vi "DelayLeft.vi"(2 "sample in":fxp<+/-,25,16>, 3 "n":i64) -> (0 "SampleOut":fxp<+/-,25,16>)   [LabVIEW 2016]
uses:
  <vilib>/rvi/Emulation/niFpgaGetClockAttributes.vi
  <vilib>/rvi/Emulation/niFpgaSctlEmulationGetInTimedLoop.vi
  <vilib>/rvi/Emulation/niFpgaEmulationReportErrorSimple.vi
  Global 1.vi
  <vilib>/rvi/Memory/Memory_Emulation/nirvimemoryFastEmulation.vi
  <vilib>/rvi/Memory/Memory_Emulation/nirvimemoryEmulation.vi
  <vilib>/rvi/Emulation/niFpgaEmulationIsFPGAContextNoSignature.vi
  <vilib>/rvi/DataTransferAndStorage/Container/Common/niFpgaContainerGetUniqueNameForEmu.vi
  <vilib>/rvi/Emulation/niFpgaProcessEmulError.vi
  <vilib>/rvi/errors/nirviReportUnexpectedCaseInternalError (U32).vi
  <vilib>/rvi/Emulation/niFpgaCriticalErrorInLSC.vi
  <vilib>/rvi/DataTransferAndStorage/Container/XNode/niFpgaContainer.xnode
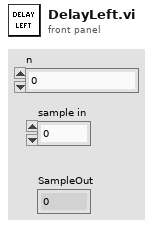
[diagram p1: front panel]
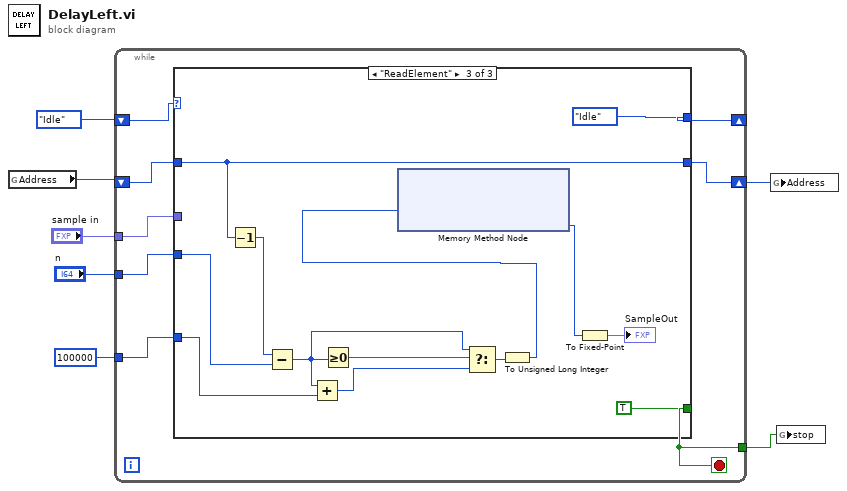
[diagram p0: block diagram]
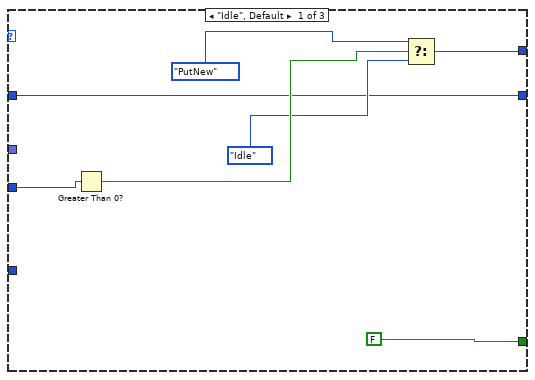
[diagram p2: hidden frame]
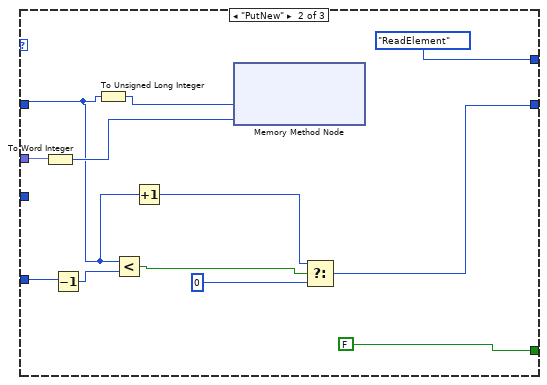
[diagram p3: hidden frame]
diagram:
  n1 = global read "Global 1.vi" "Address"() -> (w6:i64)
  n2 = while {
    shift-right: [w13] -> _
    shift-left: enum16{"Idle", "PutNew", "ReadElement"}."Idle" -> [w15]
    shift-right: [w12] -> w4
    shift-left: w6 -> [w11]
    tunnel: "n" -> [w14]
    tunnel: "sample in" -> [w10]
    tunnel: i64 100000 -> [w9]
    tunnel: [w8] -> w1
    stop <- w8 stop-if-true
    n3 = case shown="\"ReadElement\"" w15 {
      tunnel: w14 -> [w22 _ w45]
      tunnel: [w18 enum16{"Idle", "PutNew", "ReadElement"}."ReadElement" enum16{"Idle", "PutNew", "ReadElement"}."Idle"] -> w13
      tunnel: [w17 w29 w44] -> w12
      tunnel: w11 -> [w17 w23 w44]
      tunnel: w10 -> [_ w26 _]
      tunnel: w9 -> [_ w34 w43]
      tunnel: [FALSE FALSE TRUE] -> w8
      frame "Idle", Default {
        n4 = Greater Than 0?(x=w22) -> (x > 0?=w21:bool)
        n5 = Select(t=enum16{"Idle", "PutNew", "ReadElement"}."PutNew", s=w21, f=enum16{"Idle", "PutNew", "ReadElement"}."Idle") -> (s? t:f=w18:enum16{"Idle", "PutNew", "ReadElement"})
      }
      frame "PutNew" {
        n6 = To Word Integer(number=w26) -> (16bit integer=w25:i16)
        n7 = Decrement(x=w34) -> (x-1=w33:i64)
        n8 = To Unsigned Long Integer(number=w23) -> (unsigned 32bit integer=w24:u32)
        n9 = Less?(x=w23, y=w33) -> (x < y?=w31:bool)
        n10 = Increment(x=w23) -> (x+1=w32:i64)
        n11 = xnode ("Memory Method Node")("Address"=w24, "Data"=w25) -> ()  [unwired: 1 in, 1 out]
        n12 = Select(t=w32, s=w31, f=u32 0) -> (s? t:f=w29:i64)
      }
      frame "ReadElement" {
        n13 = Decrement(x=w44) -> (x-1=w46:i64)
        n14 = Subtract(x=w46, y=w45) -> (x-y=w37:i64)
        n15 = Add(x=w37, y=w43) -> (x+y=w41:i64)
        n16 = Greater Or Equal To 0?(x=w37) -> (x >= 0?=w42:bool)
        n17 = Select(t=w37, s=w42, f=w41) -> (s? t:f=w36:i64)
        n18 = To Unsigned Long Integer(number=w36) -> (unsigned 32bit integer=w35:u32)
        n19 = xnode ("Memory Method Node")("Address"=w35) -> ("Data"=w39:i16)  [unwired: 1 in, 1 out]
        n20 = To Fixed-Point(number=w39) -> (fixed-point=→"SampleOut":fxp<+/-,25,16>)  [unwired: 1 in]
      }
    }
  }
  n21 = global write "Global 1.vi" "Address"(w4) -> ()
  n22 = global write "Global 1.vi" "stop"(w1) -> ()
